vi "NegateImageAtIconIndex.vi"(8 "error in (no error)":errorcluster, 10 "Index":i32, 11 "Image Array ref in":refnum<vi>) -> (0 "error out":errorcluster, 1 "Original Image Array Value":picture[](array[picture]), 2 "New Image Array Value":picture[](array[picture]), 3 "Array ref out":refnum<vi>)   [LabVIEW 2023]
doc: "This VI accepts an Image array reference and an index and sets the Image at the index position a negative of the previous value. \n\nImage Array ref in - a reference to the image array. \nIndex - the index of the image to negate. \nArray ref out - a reference to the image array. \nNew Image array Value - the Value of the whole image array with the image at index negated. \nOriginal Image Array Value - The value of the original image array without a change."
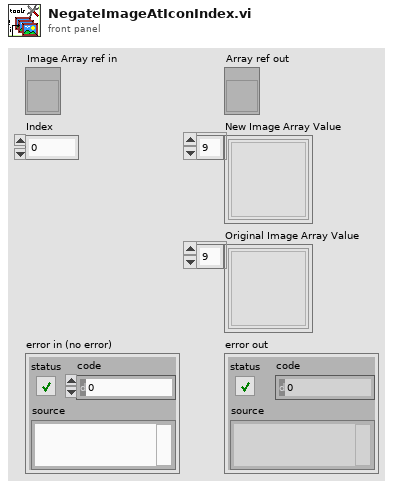
[diagram p1: front panel]
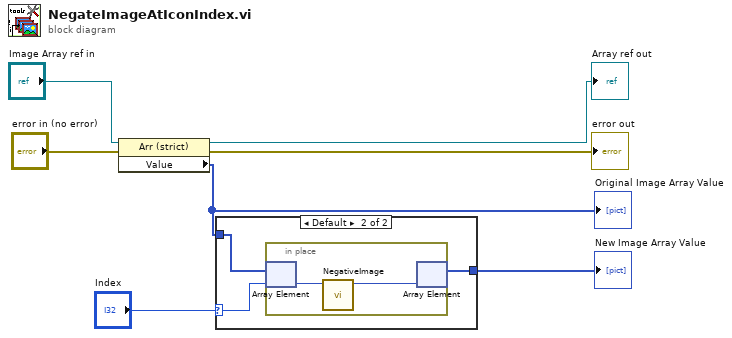
[diagram p0: block diagram]
diagram:
  n1 = property on="Property Node" class="Arr (strict)"(reference="Image Array ref in", error in="error in (no error)") -> (reference out=→"Array ref out":refnum<vi>, error out=→"error out":errorcluster, "Value"=w7:picture[])
  "Original Image Array Value" <- w7
  n2 = case shown="Default" "Index" {
    selector: "Index" -> [_ w9]
    tunnel: w7 -> [w8 w11]
    tunnel: [w8 w10] -> w6
    frame -1 {
    }
    frame Default {
      n3 = in-place "In Place Element Structure" {
        n4 = in-place-array #1(w11, w9) -> (w13:picture)
        n5 = call "NegativeImage.vi"("2D Picture in"=w13) -> ("new picture"=w12:picture)  [unwired: 10 in]
        n6 = in-place-array #1(w12) -> (w10:picture[])  [unwired: 1 out]
      }
    }
  }
  "New Image Array Value" <- w6
